vi "niRFUtil WFM Detect Edge (complex wfm).vi"(0 "Input Waveform":T3 {"y" format="%.2f"; "dx" format="%^.2e"; "x0" format="%^.2e"}, 5 "Edge Detection Settings":T1={"Mode"=enum."Sliding Window", "Sliding Window Settings"={"Chunks"=500, "Threshold (dB)"=12.0}, "Threshold Settings"={"Threshold Level (dB)"=-50.0, "Minimum Quiet Time (s)"=5e-05, "Threshold Type"=enum."Absolute"}} {"Threshold Settings"."Minimum Quiet Time (s)" format="%.3p"; "Threshold Settings"."Threshold Level (dB)" format="%.3g"; "Sliding Window Settings"."Threshold (dB)" format="%.3g"}, 7 "Edge Type":T2, 11 "error in (no error)":errorcluster) -> (4 "Output Waveform":T3 {"y" format="%.2f"; "dx" format="%^.2e"; "x0" format="%^.2e"}, 6 "Edge Detected?":bool, 8 "Detected Edge Position (s)":dbl format="%^.3e", 15 "error out":errorcluster)   [LabVIEW 2015, in "niRFUtil.lvlib"]
uses:
  niRFUtil.lvlib
  Includes/niRFUtil INC Complex Waveform.ctl
  Includes/niRFUtil INC Complex Array.ctl
  Includes/niRFUtil INC Edge Type.ctl
  Includes/niRFUtil INC Edge Detection Settings.ctl
  Measurements/niRFUtil MEAS Waveform Statistics (complex wfm).vi
  niRFUtil WFM Parse Waveform - Duration (complex wfm).vi
  Conversion/niRFUtil CONV 1 Ohm Voltage to dBm (complex wfm).vi
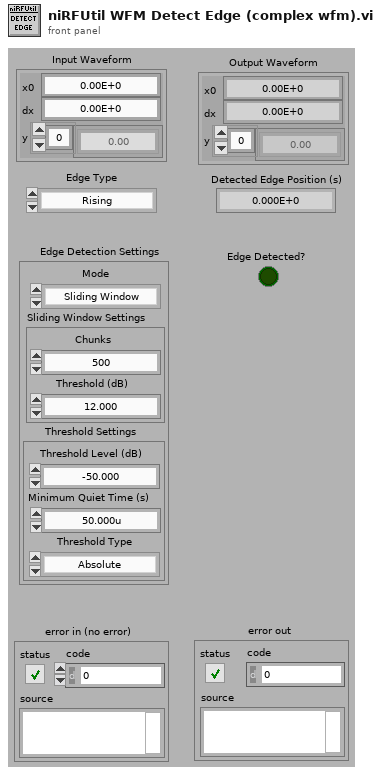
[diagram p1: front panel]
types:
  T1 = typedef "niRFUtil.lvlib/niRFUtil INC Edge Detection Settings.ctl" = cluster{"Mode":enum16{"Sliding Window", "Threshold"}, "Sliding Window Settings":cluster{"Chunks":i32, "Threshold (dB)":dbl}, "Threshold Settings":cluster{"Threshold Level (dB)":dbl, "Minimum Quiet Time (s)":dbl, "Threshold Type":enum16{"Relative", "Absolute"}}}
  T2 = typedef "niRFUtil.lvlib/niRFUtil INC Edge Type.ctl" = enum16{"Rising", "Falling"}
  T3 = typedef "niRFUtil.lvlib/niRFUtil INC Complex Waveform.ctl" = cluster{"x0":dbl, "dx":dbl, "y":T4}
  T4 = typedef "niRFUtil.lvlib/niRFUtil INC Complex Array.ctl" = csg[]
  T5 = cluster{"Threshold Level (dB)":dbl, "Minimum Quiet Time (s)":dbl, "Threshold Type":enum16{"Relative", "Absolute"}}
  T6 = typedef "niRFUtil.lvlib/niRFUtil INC Real Waveform.ctl" = cluster{"x0":dbl, "dx":dbl, "y":T7}
  T7 = typedef "niRFUtil.lvlib/niRFUtil INC Real Array.ctl" = sgl[]
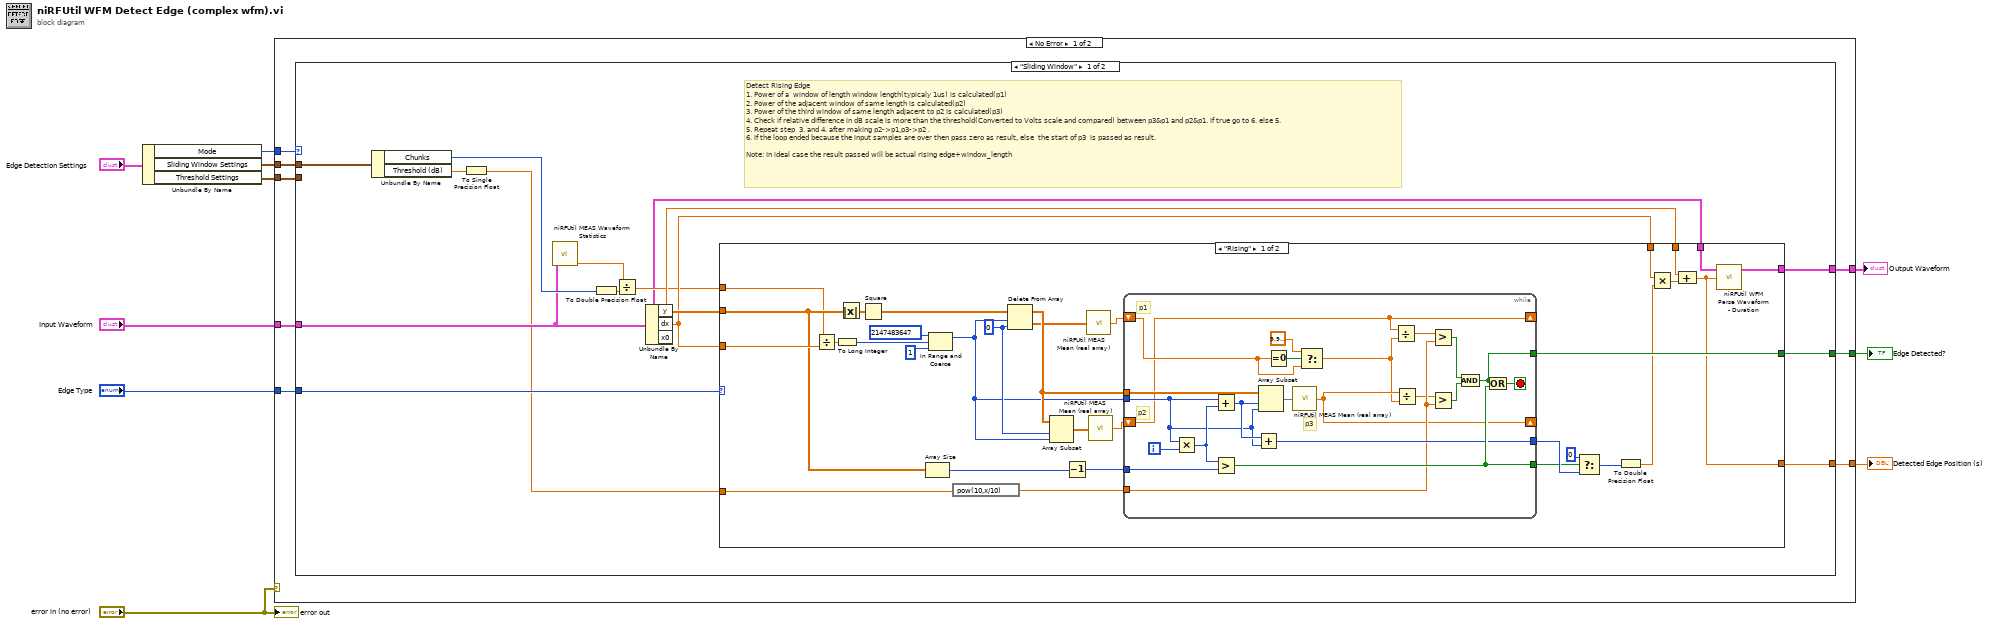
[diagram p0: block diagram]
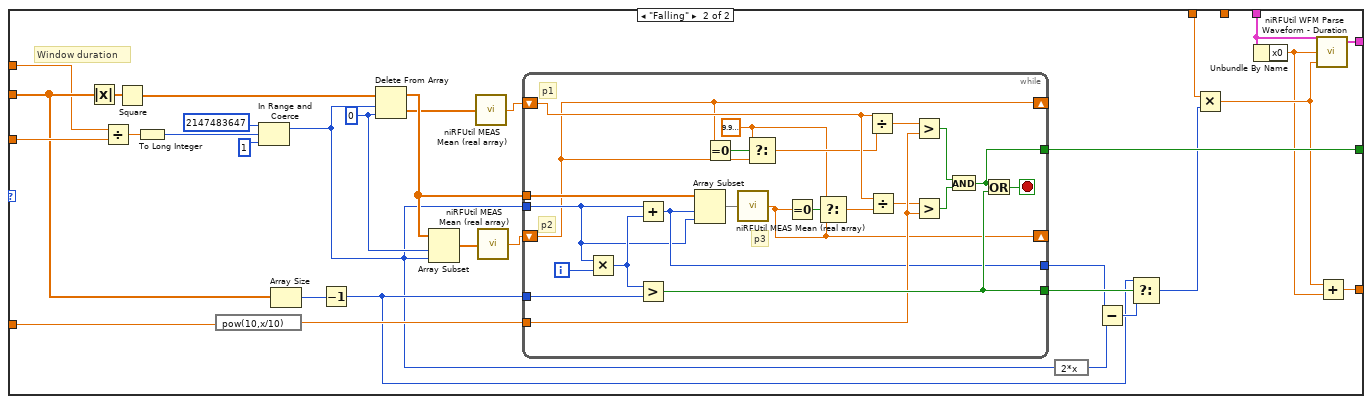
[diagram p2: hidden frame]
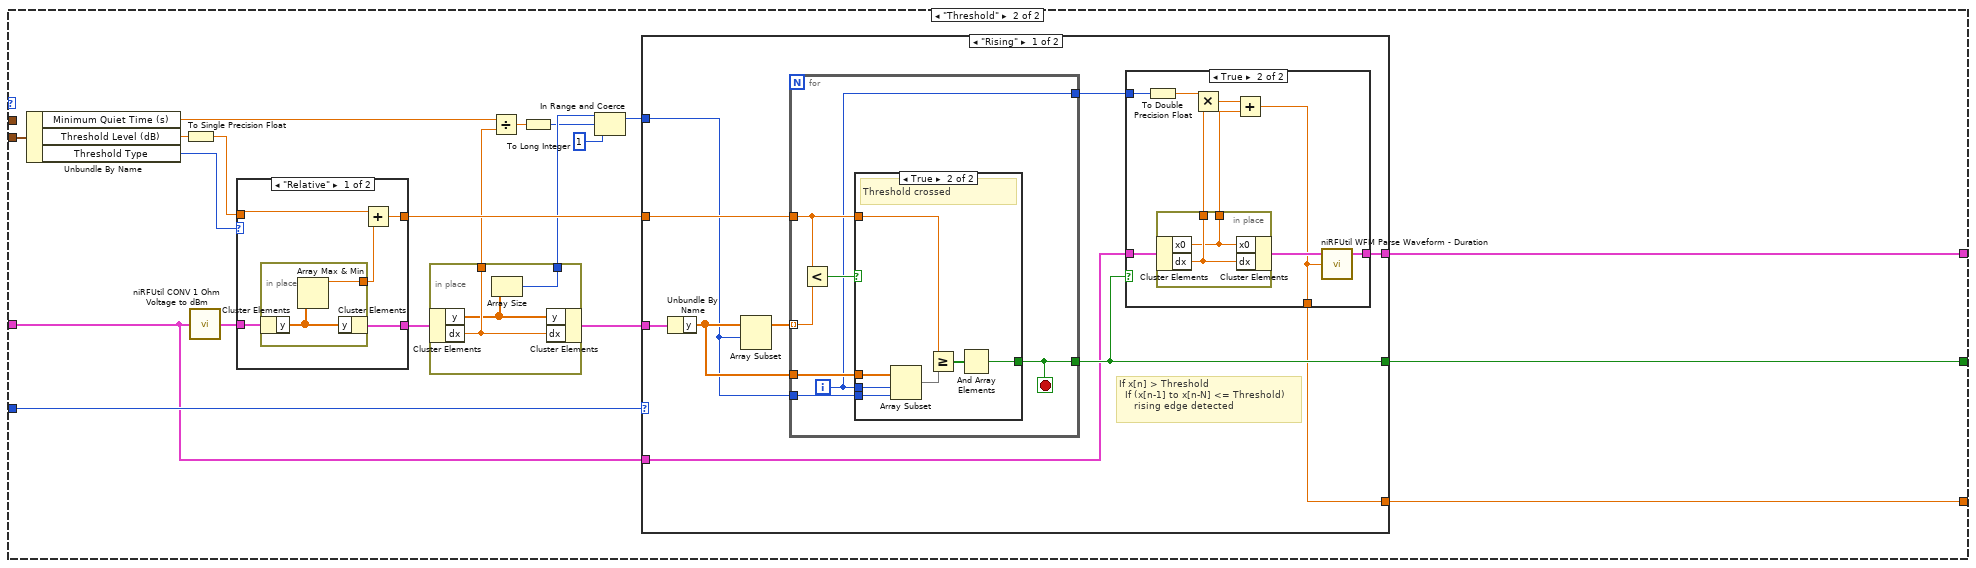
[diagram p3: hidden frame]
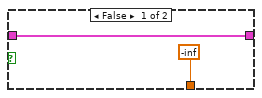
[diagram p4: hidden frame]
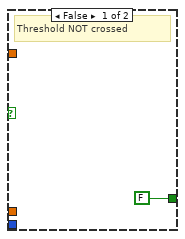
[diagram p5: hidden frame]
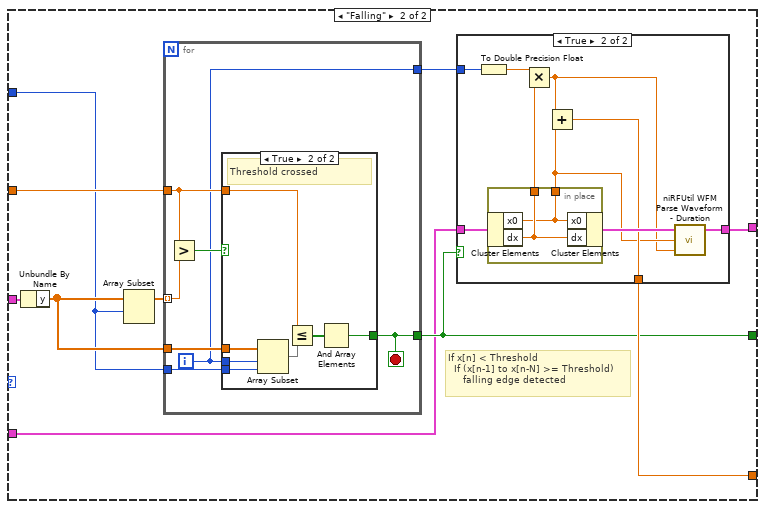
[diagram p6: hidden frame]
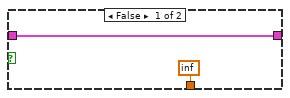
[diagram p7: hidden frame]
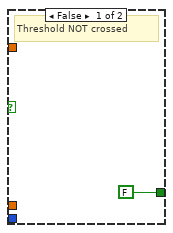
[diagram p8: hidden frame]
diagram:
  n1 = Unbundle By Name("Edge Detection Settings") -> ("Mode"=w3:enum16{"Sliding Window", "Threshold"}, "Sliding Window Settings"=w2:cluster{"Chunks":i32, "Threshold (dB)":dbl}, "Threshold Settings"=w1:T5)
  n2 = case shown="No Error" "error in (no error)" {
    tunnel: [w18 _] -> w10
    tunnel: [w17 _] -> w9
    tunnel: "Edge Type" -> [w16 _]
    tunnel: [w15 _] -> w7
    tunnel: "Input Waveform" -> [w14 _]
    tunnel: w3 -> [w13 _]
    tunnel: w2 -> [w12 _]
    tunnel: w1 -> [w11 _]
    frame No Error {
      n3 = case shown="\"Sliding Window\"" w13 {
        tunnel: [w33 w147] -> w18
        tunnel: [w31 w145] -> w17
        tunnel: w16 -> [w30 w158]
        tunnel: [w27 w146] -> w15
        tunnel: w14 -> [w21 w144]
        tunnel: w12 -> [w24 _]
        tunnel: w11 -> [_ w161]
        frame "Sliding Window" {
          # "Detect Rising Edge\n1. Power of a  window of length window length(typicaly 1us) is calculated(p1)\n2. Power of the adjacent window of same length is calculated(p2)\n3. Power of the third window of same length adjacent to p2 is calculated(p3)\n4. Check if relative difference in dB scale is more than the threshold(Converted to Volts scale and compared) between p3&p1 and p2&p1. If true go to 6. else 5.\n5. Repeat step  3. and 4. after making p2->p1,p3->p2 .\n6. If the loop ended because the input samples are over then pass zero as result, else  the start of p3  is passed as result.\n\nNote: In ideal case the result passed will be actual rising edge+window_length"
          n4 = Unbundle By Name(w24) -> ("Chunks"=w23:i32, "Threshold (dB)"=w22:dbl)
          n5 = To Single Precision Float(number=w22) -> (single precision float=w19:sgl)
          n6 = call-poly "niRFUtil MEAS Waveform Statistics.vi"("Waveform In"=w21) -> ("Duration"=w26:dbl)  [unwired: 4 in, 3 out]
          n7 = To Double Precision Float(number=w23) -> (double precision float=w20:dbl)
          n8 = Divide(x=w26, y=w20) -> (x/y=w25:dbl)
          n9 = Unbundle By Name(w21) -> ("y"=w32:T4, "dx"=w29:dbl, "x0"=w28:dbl)
          n10 = case shown="\"Rising\"" w30 {
            tunnel: [w39 w94] -> w31
            tunnel: w29 -> [w65 w119]
            tunnel: w32 -> [w64 w118]
            tunnel: [w63 w117] -> w33
            tunnel: w25 -> [w62 w116]
            tunnel: w19 -> [w61 w115]
            tunnel: w29 -> [w44 w101]
            tunnel: w28 -> [w43 _]
            tunnel: w21 -> [w42 w99]
            tunnel: [w41 w102] -> w27
            frame "Rising" {
              w54 = 0 ("index")
              n11 = Divide(x=w62, y=w65) -> (x/y=w59:dbl)
              n12 = To Long Integer(number=w59) -> (32bit integer=w37:i32)
              n13 = Absolute Value(x=w64) -> (abs(x)=w49:sgl[])
              n14 = Square(x=w49) -> (x^2=w58:sgl[])
              n15 = Array Size(array=w64) -> (size(s)=w50:i32)
              n16 = In Range and Coerce(upper limit=2147483647, x=w37, lower limit=1) -> (coerced(x)=w34:i32)  [unwired: 1 out]
              n17 = expression code="pow(10,x/10)"(w61) -> (w53:sgl)
              n18 = Delete From Array(array=w58, length=w34, index=w54) -> (deleted portion=w52:sgl[], array with subset deleted=w55:sgl[])
              n19 = Array Subset(array=w55, index=w54, length=w34) -> (w56:sgl[])
              n20 = Decrement(x=w50) -> (x-1=w51:i32)
              n21 = call "niRFUtil MEAS Mean (real array).vi"("Real Array"=w52) -> ("Mean"=w46:sgl)  [unwired: 14 in]
              n22 = call "niRFUtil MEAS Mean (real array).vi"("Real Array"=w56) -> ("Mean"=w57:sgl)  [unwired: 14 in]
              n23 = while {
                tunnel: [w80] -> w48
                tunnel: [w86] -> w47
                tunnel: w51 -> [w85]
                tunnel: w55 -> [w83]
                shift-right: [w67] -> _
                shift-left: w46 -> [w68]
                tunnel: w53 -> [w77]
                tunnel: w34 -> [w69]
                shift-right: [w72] -> _
                shift-left: w57 -> [w67]
                tunnel: [w66] -> w63
                i -> [w76]
                stop <- w87 stop-if-true
                # "p3"
                # "p1"
                # "p2"
                n24 = Multiply(x=w69, y=w76) -> (x*y=w71:i32)
                n25 = Add(x=w69, y=w71) -> (x+y=w75:i32)
                n26 = Greater?(x=w71, y=w85) -> (0:w86:bool)
                n27 = Add(x=w75, y=w69) -> (x+y=w80:i32)
                n28 = Array Subset(array=w83, index=w75, length=w69) -> (w84:sgl[])
                n29 = Equal To 0?(x=w68) -> (x = 0?=w79:bool)
                n30 = call "niRFUtil MEAS Mean (real array).vi"("Real Array"=w84) -> ("Mean"=w72:sgl)  [unwired: 14 in]
                n31 = Select(t=sgl 1e-06, s=w79, f=w68) -> (s? t:f=w70:sgl)
                n32 = Divide(x=w67, y=w70) -> (x/y=w73:sgl)
                n33 = Divide(x=w72, y=w70) -> (x/y=w74:sgl)
                n34 = Greater?(x=w73, y=w77) -> (0:w82:bool)
                n35 = Greater?(x=w74, y=w77) -> (0:w81:bool)
                n36 = And(x=w82, y=w81) -> (x .and. y?=w66:bool)
                n37 = Or(x=w66, y=w86) -> (x .or. y?=w87:bool)
              }
              n38 = Select(t=0, s=w47, f=w48) -> (s? t:f=w40:i32)
              n39 = To Double Precision Float(number=w40) -> (double precision float=w38:dbl)
              n40 = Multiply(x=w44, y=w38) -> (x*y=w45:dbl)
              n41 = Compound Arithmetic op=ADD(w43, w45) -> (w39:dbl)
              n42 = call-poly "niRFUtil WFM Parse Waveform - Duration.vi"("Start (-Inf)"=w39, "Waveform In"=w42) -> ("Waveform Out"=w41:T3)  [unwired: 3 in]
            }
            frame "Falling" {
              w109 = 0 ("index")
              # "Window duration"
              n43 = Absolute Value(x=w118) -> (abs(x)=w105:sgl[])
              n44 = Divide(x=w116, y=w119) -> (x/y=w114:dbl)
              n45 = Square(x=w105) -> (x^2=w113:sgl[])
              n46 = To Long Integer(number=w114) -> (32bit integer=w89:i32)
              n47 = expression code="pow(10,x/10)"(w115) -> (w108:sgl)
              n48 = In Range and Coerce(upper limit=2147483647, x=w89, lower limit=1) -> (coerced(x)=w88:i32)  [unwired: 1 out]
              n49 = Array Size(array=w118) -> (size(s)=w106:i32)
              n50 = Decrement(x=w106) -> (x-1=w95:i32)
              n51 = Delete From Array(array=w113, length=w88, index=w109) -> (deleted portion=w107:sgl[], array with subset deleted=w110:sgl[])
              n52 = Array Subset(array=w110, index=w109, length=w88) -> (w111:sgl[])
              n53 = call "niRFUtil MEAS Mean (real array).vi"("Real Array"=w107) -> ("Mean"=w103:sgl)  [unwired: 14 in]
              n54 = call "niRFUtil MEAS Mean (real array).vi"("Real Array"=w111) -> ("Mean"=w112:sgl)  [unwired: 14 in]
              n55 = while {
                tunnel: [w132] -> w97
                tunnel: [w141] -> w104
                tunnel: w95 -> [w140]
                tunnel: w110 -> [w138]
                shift-right: [w125] -> _
                shift-left: w103 -> [w126]
                tunnel: w108 -> [w134]
                tunnel: w88 -> [w127]
                shift-right: [w122] -> _
                shift-left: w112 -> [w125]
                tunnel: [w129] -> w117
                i -> [w133]
                stop <- w142 stop-if-true
                w120 = sgl 1e-06 ("t")
                # "p3"
                # "p1"
                # "p2"
                n56 = Multiply(x=w127, y=w133) -> (x*y=w128:i32)
                n57 = Add(x=w127, y=w128) -> (x+y=w132:i32)
                n58 = Greater?(x=w128, y=w140) -> (0:w141:bool)
                n59 = Array Subset(array=w138, index=w132, length=w127) -> (w139:sgl[])
                n60 = Equal To 0?(x=w125) -> (x = 0?=w135:bool)
                n61 = call "niRFUtil MEAS Mean (real array).vi"("Real Array"=w139) -> ("Mean"=w122:sgl)  [unwired: 14 in]
                n62 = Select(t=w120, s=w135, f=w125) -> (s? t:f=w124:sgl)
                n63 = Equal To 0?(x=w122) -> (x = 0?=w123:bool)
                n64 = Select(t=w120, s=w123, f=w122) -> (s? t:f=w121:sgl)
                n65 = Divide(x=w126, y=w124) -> (x/y=w130:sgl)
                n66 = Divide(x=w126, y=w121) -> (x/y=w131:sgl)
                n67 = Greater?(x=w130, y=w134) -> (0:w137:bool)
                n68 = Greater?(x=w131, y=w134) -> (0:w136:bool)
                n69 = And(x=w137, y=w136) -> (x .and. y?=w129:bool)
                n70 = Or(x=w129, y=w141) -> (x .or. y?=w142:bool)
              }
              n71 = expression code="2*x"(w88) -> (w98:i32)
              n72 = Subtract(x=w97, y=w98) -> (x-y=w96:i32)
              n73 = Select(t=w95, s=w104, f=w96) -> (s? t:f=w100:i32)
              n74 = Multiply(x=w101, y=w100) -> (x*y=w93:dbl)
              n75 = Unbundle By Name(w99) -> ("x0"=w92:dbl)
              n76 = call-poly "niRFUtil WFM Parse Waveform - Duration.vi"("Duration (Inf)"=w93, "Start (-Inf)"=w92, "Waveform In"=w99) -> ("Waveform Out"=w102:T3)  [unwired: 2 in]
              n77 = Add(x=w93, y=w92) -> (x+y=w94:dbl)
            }
          }
        }
        frame "Threshold" {
          n78 = Unbundle By Name(w161) -> ("Minimum Quiet Time (s)"=w153:dbl, "Threshold Level (dB)"=w160:dbl, "Threshold Type"=w159:enum16{"Relative", "Absolute"})
          n79 = To Single Precision Float(number=w160) -> (single precision float=w143:sgl)
          n80 = call-poly "niRFUtil CONV 1 Ohm Voltage to dBm.vi"("Complex Waveform (V)"=w144) -> ("Real Waveform (dBm)"=w162:T6)  [unwired: 14 in]
          n81 = case shown="\"Relative\"" w159 {
            tunnel: w162 -> [w246 w249]
            tunnel: [w244 w249] -> w156
            tunnel: [w243 w250] -> w157
            tunnel: w143 -> [w242 w250]
            frame "Relative" {
              n82 = in-place {
                in-place-border: [w247] -> w245
                n83 = in-place-cluster #1(w246) -> ("y"=w248:T7)
                n84 = Array Max & Min(array=w248) -> (max value=w247:sgl)  [unwired: 3 out]
                n85 = in-place-cluster #1("y"=w248) -> (w244:T6)
              }
              n86 = Add(x=w242, y=w245) -> (x+y=w243:sgl)
            }
            frame "Absolute" {
            }
          }
          n87 = in-place {
            in-place-border: [w165] -> w154
            in-place-border: [w163] -> w150
            n88 = in-place-cluster #2(w156) -> ("y"=w164:T7, "dx"=w165:dbl)
            n89 = Array Size(array=w164) -> (size(s)=w163:i32)
            n90 = in-place-cluster #2("y"=w164, "dx"=w165) -> (w155:T6)
          }
          n91 = Divide(x=w153, y=w154) -> (x/y=w152:dbl)
          n92 = To Long Integer(number=w152) -> (32bit integer=w149:i32)
          n93 = In Range and Coerce(upper limit=w150, x=w149, lower limit=1) -> (coerced(x)=w148:i32)  [unwired: 1 out]
          n94 = case shown="\"Rising\"" w158 {
            tunnel: w155 -> [w171 w209]
            tunnel: w157 -> [w175 w213]
            tunnel: w148 -> [w172 w204]
            tunnel: [w169 w206] -> w147
            tunnel: [w170 w207] -> w146
            tunnel: [w167 w208] -> w145
            tunnel: w144 -> [w166 w205]
            frame "Rising" {
              # "If x[n] > Threshold\n  If (x[n-1] to x[n-N] <= Threshold)\n     rising edge detected"
              n95 = Unbundle By Name(w171) -> ("y"=w174:T7)
              n96 = Array Subset(array=w174, index=w172) -> (w173:T7)  [unwired: 1 in]
              n97 = for {
                tunnel: w173 -> [w195] mode=indexing
                tunnel: w175 -> [w191]
                tunnel: w174 -> [w193]
                tunnel: w172 -> [w192]
                tunnel: [w190] -> w169
                tunnel: [w189] -> w168
                i -> [w189]
                stop <- w190 stop-if-true
                n98 = Less?(x=w191, y=w195) -> (x < y?=w194:bool)
                n99 = case shown="True" w194 {
                  tunnel: w193 -> [_ w203]
                  tunnel: w189 -> [_ w202]
                  tunnel: w192 -> [_ w201]
                  tunnel: w191 -> [_ w200]
                  tunnel: [FALSE w197] -> w190
                  frame False {
                    # "Threshold NOT crossed"
                  }
                  frame True {
                    # "Threshold crossed"
                    n100 = Array Subset(array=w203, index=w202, length=w201) -> (w199:T7)
                    n101 = Greater Or Equal?(x=w200, y=w199) -> (x >= y?=w198:bool[])
                    n102 = And Array Elements(Boolean array=w198) -> (logical AND=w197:bool)
                  }
                }
              }
              n103 = case shown="True" w169 {
                tunnel: w166 -> [w177 w185]
                tunnel: [w177 w186] -> w170
                tunnel: w168 -> [_ w183]
                tunnel: [-inf w179] -> w167
                frame False {
                }
                frame True {
                  n104 = To Double Precision Float(number=w183) -> (double precision float=w178:dbl)
                  n105 = in-place {
                    in-place-border: [w188] -> w182
                    in-place-border: [w187] -> w180
                    n106 = in-place-cluster #3(w185) -> ("x0"=w187:dbl, "dx"=w188:dbl)
                    n107 = in-place-cluster #3("x0"=w187, "dx"=w188) -> (w184:T3)
                  }
                  n108 = Multiply(x=w178, y=w182) -> (x*y=w181:dbl)
                  n109 = Add(x=w181, y=w180) -> (x+y=w179:dbl)
                  n110 = call-poly "niRFUtil WFM Parse Waveform - Duration.vi"("Start (-Inf)"=w179, "Waveform In"=w184) -> ("Waveform Out"=w186:T3)  [unwired: 3 in]
                }
              }
            }
            frame "Falling" {
              # "If x[n] < Threshold\n  If (x[n-1] to x[n-N] >= Threshold)\n     falling edge detected"
              n111 = Unbundle By Name(w209) -> ("y"=w212:T7)
              n112 = Array Subset(array=w212, index=w204) -> (w211:T7)  [unwired: 1 in]
              n113 = for {
                tunnel: w211 -> [w233] mode=indexing
                tunnel: w213 -> [w229]
                tunnel: w212 -> [w231]
                tunnel: w204 -> [w230]
                tunnel: [w228] -> w206
                tunnel: [w227] -> w210
                i -> [w227]
                stop <- w228 stop-if-true
                n114 = Greater?(x=w229, y=w233) -> (0:w232:bool)
                n115 = case shown="True" w232 {
                  tunnel: w231 -> [_ w241]
                  tunnel: w227 -> [_ w240]
                  tunnel: w230 -> [_ w239]
                  tunnel: w229 -> [_ w238]
                  tunnel: [FALSE w235] -> w228
                  frame False {
                    # "Threshold NOT crossed"
                  }
                  frame True {
                    # "Threshold crossed"
                    n116 = Array Subset(array=w241, index=w240, length=w239) -> (w237:T7)
                    n117 = Less Or Equal?(x=w238, y=w237) -> (x <= y?=w236:bool[])
                    n118 = And Array Elements(Boolean array=w236) -> (logical AND=w235:bool)
                  }
                }
              }
              n119 = case shown="True" w206 {
                tunnel: w205 -> [w215 w223]
                tunnel: [w215 w224] -> w207
                tunnel: w210 -> [_ w221]
                tunnel: [inf w219] -> w208
                frame False {
                }
                frame True {
                  n120 = To Double Precision Float(number=w221) -> (double precision float=w218:dbl)
                  n121 = in-place {
                    in-place-border: [w226] -> w220
                    in-place-border: [w225] -> w217
                    n122 = in-place-cluster #4(w223) -> ("x0"=w225:dbl, "dx"=w226:dbl)
                    n123 = in-place-cluster #4("x0"=w225, "dx"=w226) -> (w222:T3)
                  }
                  n124 = Multiply(x=w218, y=w220) -> (x*y=w216:dbl)
                  n125 = Add(x=w216, y=w217) -> (x+y=w219:dbl)
                  n126 = call-poly "niRFUtil WFM Parse Waveform - Duration.vi"("Duration (Inf)"=w216, "Start (-Inf)"=w217, "Waveform In"=w222) -> ("Waveform Out"=w224:T3)  [unwired: 2 in]
                }
              }
            }
          }
        }
      }
    }
    frame Error {
    }
  }
  "Detected Edge Position (s)" <- w9
  "Edge Detected?" <- w10
  "Output Waveform" <- w7
  "error out" <- "error in (no error)"
